vi "Autonomous.vi"   [LabVIEW 2019]
doc: "This VI starts when autonomous period begins, and will automatically be terminated when it ends. You can carry out timed or sensor driven operations directly to I/O or to subsystems without needing to return to the caller."
uses:
  <vilib>/Rock Robotics/Network Tables/NT Read String.vi
  Framework/Robot Global Data.vi
types:
  T1 = typedef "Auto Controls.ctl" = cluster{"Drive Duration":dbl, "Left Speed":dbl, "Right Speed":dbl, "Set Point":dbl, "Set Point Duration":dbl, "Command":enum16{"", "Drive Forwards", "Drive Backwards", "Stop", "Turn Left", "Turn Right", "Drop Intake", "Lift Intake", "Intake", "Shooter", "Transfer", "Wait"}, "Wait ms":dbl}[]
  T2 = typedef "Command Status Info.ctl" = cluster{"Name":string, "Status":T3, "notifier out":T4}
  T3 = typedef "Completion Status.ctl" = enum16{"Successful", "Aborted", "Incomplete"}
  T4 = typedef "Completion Notifier.ctl" = refnum<notifier>
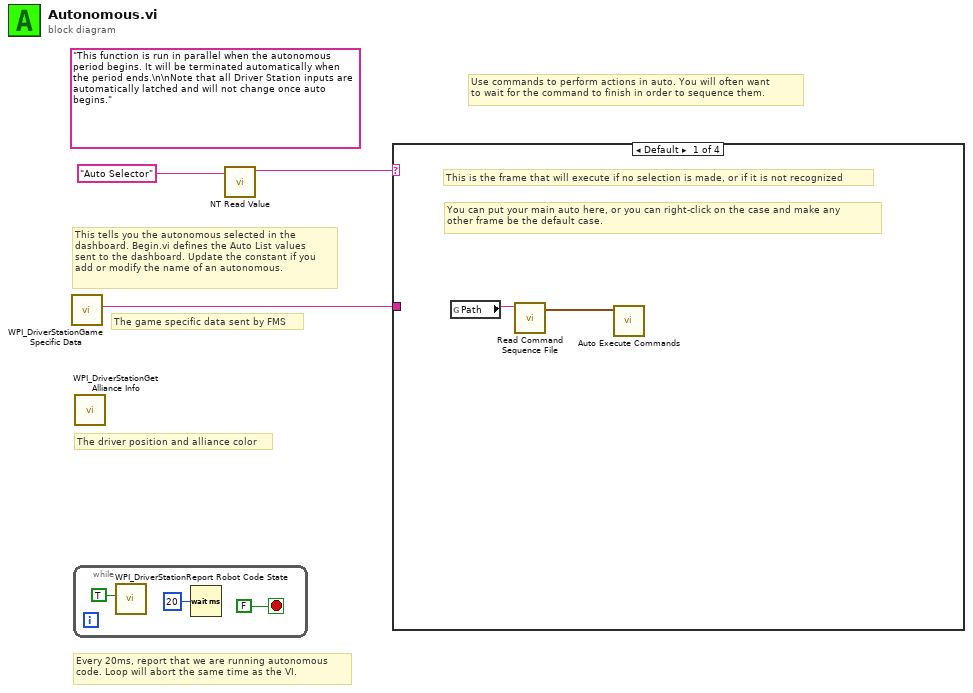
[diagram p0: block diagram]
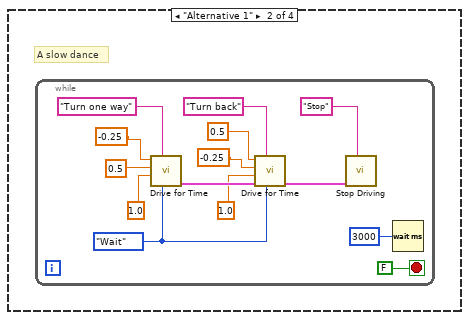
[diagram p2: hidden frame]
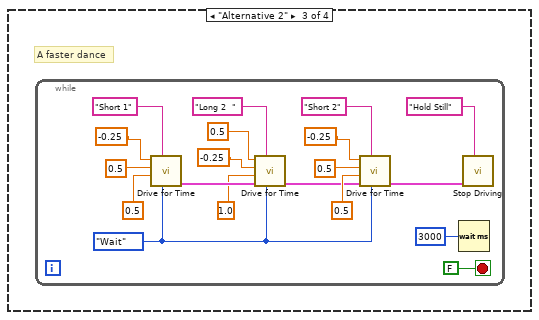
[diagram p3: hidden frame]
diagram:
  (unwired) "This function is run in parallel when the autonomous period begins. It will be terminated automatically when the period ends.\n\nNote that all Driver Station inputs are automatically latched and will not change once auto begins."
  # "The game specific data sent by FMS"
  # "This tells you the autonomous selected in the \ndashboard. Begin.vi defines the Auto List values\nsent to the dashboard. Update the constant if you\nadd or modify the name of an autonomous."
  # "Every 20ms, report that we are running autonomous\ncode. Loop will abort the same time as the VI."
  # "Use commands to perform actions in auto. You will often want\nto wait for the command to finish in order to sequence them."
  # "The driver position and alliance color"
  n1 = call <vilib>:"WPI_DriverStationGame Specific Data.vi"() -> ("Game Specific Data"=w1:string)  [unwired: 11 in]
  n2 = while {
    stop <- FALSE stop-if-true
    n3 = call <vilib>:"WPI_DriverStationReport Robot Code State.vi"("Autonomous"=TRUE) -> ()  [unwired: 10 in, 1 out]
    n4 = Wait (ms)(milliseconds to wait=u32 20) -> ()  [unwired: 1 out]
  }
  n5 = call <vilib>:"WPI_DriverStationGet Alliance Info.vi"() -> ()  [unwired: 12 out]
  n6 = call-poly <vilib>:"NT Read Value.vi"("Name"="Auto Selector") -> ("String"=w2:string)  [unwired: 9 in, 1 out]
  n7 = case shown="Default" w2 {
    tunnel: w1 -> [_ _ _ _]
    frame Default {
      # "You can put your main auto here, or you can right-click on the case and make any\nother frame be the default case."
      # "This is the frame that will execute if no selection is made, or if it is not recognized"
      n8 = global read "Robot Global Data.vi" "Path"() -> (w7:string)
      n9 = call "Read Command Sequence File.vi"("Path Name"=w7) -> ("Auto Commands"=w8:T1)  [unwired: 10 in]
      n10 = call "Auto Execute Commands.vi"("Auto Commands"=w8) -> ()  [unwired: 11 in]
    }
    frame "Alternative 1" {
      # "A slow dance"
      n11 = while {
        stop <- FALSE stop-if-true
        w13 = enum16{"Start", "Wait"}."Wait" ("Synchronication")
        n12 = call "Drive for Time.vi"("Synchronization"=w13, "Description"="Turn one way", "Seconds"=1.0 ("Delay (s)"), "Right Speed"=0.5 ("X axis value"), "Left Speed"=-0.25 ("X axis value")) -> ("Command Info Out"=w22:T2)  [unwired: 6 in]
        n13 = call "Drive for Time.vi"("Synchronization"=w13, "Description"="Turn back", "Command Info In"=w22, "Seconds"=1.0 ("Delay (s)"), "Right Speed"=-0.25 ("X axis value"), "Left Speed"=0.5 ("X axis value")) -> ("Command Info Out"=w12:T2)  [unwired: 5 in]
        n14 = call "Stop Driving.vi"("Description"="Stop", "Command Info In"=w12) -> ()  [unwired: 9 in, 1 out]
        n15 = Wait (ms)(milliseconds to wait=u32 3000 ("millisecond timer value")) -> ()  [unwired: 1 out]
      }
    }
    frame "Alternative 2" {
      # "A faster dance"
      n16 = while {
        stop <- FALSE stop-if-true
        w23 = enum16{"Start", "Wait"}."Wait" ("Synchronication")
        n17 = call "Drive for Time.vi"("Synchronization"=w23, "Description"="Short 1", "Seconds"=0.5 ("Delay (s)"), "Right Speed"=0.5 ("X axis value"), "Left Speed"=-0.25 ("X axis value")) -> ("Command Info Out"=w41:T2)  [unwired: 6 in]
        n18 = call "Drive for Time.vi"("Synchronization"=w23, "Description"="Long 2  ", "Command Info In"=w41, "Seconds"=1.0 ("Delay (s)"), "Right Speed"=-0.25 ("X axis value"), "Left Speed"=0.5 ("X axis value")) -> ("Command Info Out"=w25:T2)  [unwired: 5 in]
        n19 = call "Drive for Time.vi"("Synchronization"=w23, "Description"="Short 2", "Command Info In"=w25, "Seconds"=0.5 ("Delay (s)"), "Right Speed"=0.5 ("X axis value"), "Left Speed"=-0.25 ("X axis value")) -> ("Command Info Out"=w24:T2)  [unwired: 5 in]
        n20 = Wait (ms)(milliseconds to wait=u32 3000 ("millisecond timer value")) -> ()  [unwired: 1 out]
        n21 = call "Stop Driving.vi"("Description"="Hold Still", "Command Info In"=w24) -> ()  [unwired: 9 in, 1 out]
      }
    }
    frame "Your Turn" {
    }
  }
